vi "Register Settings Changes.vi"(8 "error in (no error)":errorcluster, 10 "Settings Data":T1, 11 "VIStore in":refnum<class "VIStore.lvclass">) -> (0 "error out":errorcluster, 3 "VIStore out":refnum<class "VIStore.lvclass">)   [LabVIEW 2015, in "VI App Store.lvlib" / "VIStore.lvclass"]
uses:
  VIStore.lvclass
  Classes/Settings Item/Settings Data.ctl
  VIStore.lvclass/VIStore.ctl
  Classes/Settings Item/Settings.lvclass
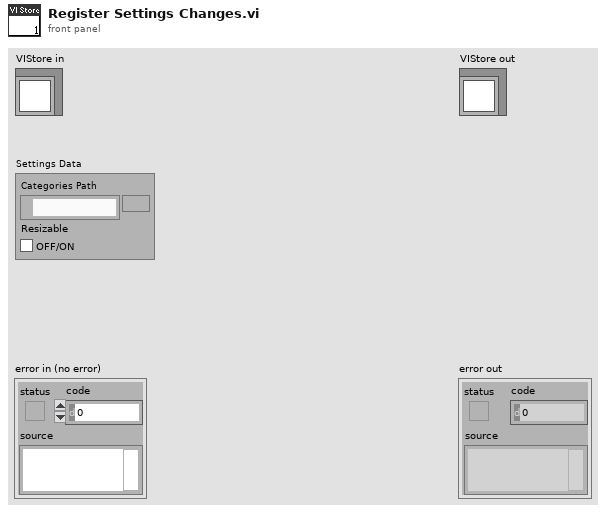
[diagram p1: front panel]
types:
  T1 = typedef "Item Actor.lvlib/Settings.lvclass/Settings Data.ctl" = cluster{"Categories Path":path, "Resizable":bool}
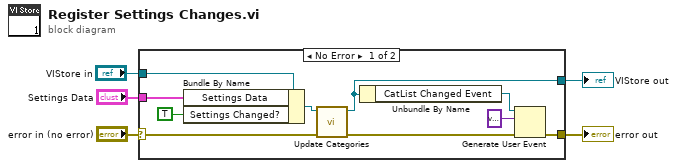
[diagram p0: block diagram]
diagram:
  n1 = case shown="No Error" "error in (no error)" {
    selector: "error in (no error)" -> [w12 w17]
    tunnel: [w8 w17] -> w4
    tunnel: [w7 w16] -> w2
    tunnel: "VIStore in" -> [w15 w16]
    tunnel: "Settings Data" -> [w14 _]
    frame No Error {
      n2 = Bundle By Name(cluster=w15, "Settings Data"=w14, "Settings Changed?"=TRUE) -> (w13:refnum<class "VIStore.lvclass">)
      n3 = call "Update Categories.vi"("error in (no error)"=w12, "VIStore in"=w13) -> ("error out"=w9:errorcluster, "VIStore out"=w7:refnum<class "VIStore.lvclass">)  [unwired: 8 in]
      n4 = Unbundle By Name(w7) -> ("CatList Changed Event"=w11:refnum<user-event>)
      n5 = Generate User Event(user event=w11, event data cluster=variant ("event data"), error in=w9) -> (error out=w8:errorcluster)  [unwired: 1 in, 1 out]
    }
    frame Error {
    }
  }
  "error out" <- w4
  "VIStore out" <- w2
